vi "to8bits.vi"(2 "error in (no error)":errorcluster, 3 "Image":T1) -> (0 "error out":errorcluster, 1 "Image":T1)   [LabVIEW 2009]
uses:
  <vilib>/vision/Image Controls.llb/IMAQ Image.ctl
  <vilib>/vision/NI_Vision_Development_Module.lvlib
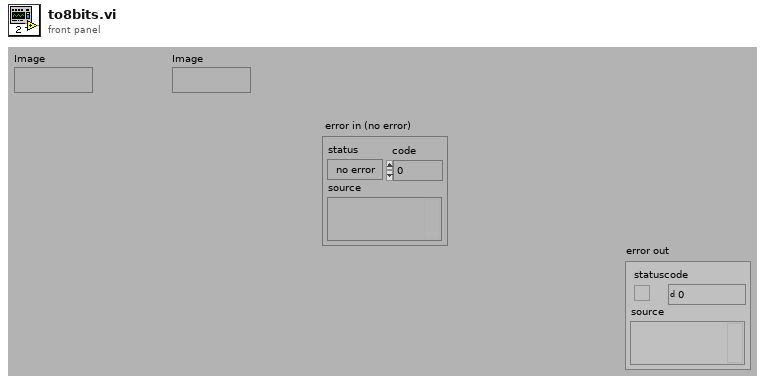
[diagram p1: front panel]
types:
  T1 = typedef "IMAQ Image.ctl" = refnum<image>
  T2 = cluster{"Mean Value":sgl, "Standard Variation":sgl, "Minimal Value":sgl, "Maximal Value":sgl, "Area (calibrated)":sgl, "Area (pixels)":i32, "%":sgl}
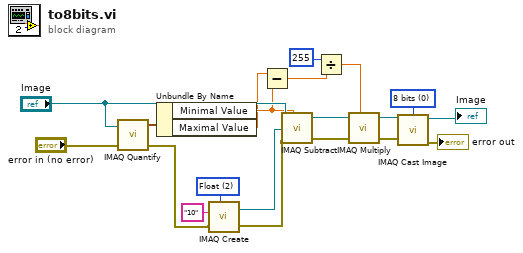
[diagram p0: block diagram]
diagram:
  w8 = u32 2 items=["8 bits", "16 bits", "Float", "Complex", "RGB", "HSL"] ("Image Type")
  w10 = u32 0 items=["8 bits", "16 bits", "Float", "Complex", "RGB", "HSL"] ("Image Type")
  n1 = call "IMAQ Quantify"("error in (no error)"="error in (no error)", "Image"="Image") -> ("error out"=w5:errorcluster, "Global Report"=w18:T2)  [unwired: 1 in, 1 out]
  n2 = Unbundle By Name(w18) -> ("Minimal Value"=w17:sgl, "Maximal Value"=w16:sgl)
  n3 = call "IMAQ Create"("Image Name"="10", "Image Type"=w8, "error in (no error)"=w5) -> ("New Image"=w7:T1, "error out"=w4:errorcluster)  [unwired: 2 in]
  n4 = Subtract(x=w16, y=w17) -> (x-y=w14:sgl)
  n5 = call "IMAQ Subtract"("Image Src A"="Image", "Constant"=w17, "Image Dst"=w7, "error in (no error)"=w4) -> ("Image Dst Out"=w13:T1, "error out"=w3:errorcluster)  [unwired: 3 in]
  n6 = Divide(x=u16 255, y=w14) -> (x/y=w12:sgl)
  n7 = call "IMAQ Multiply"("Image Src A"=w13, "Constant"=w12, "error in (no error)"=w3) -> ("Image Dst Out"=w11:T1, "error out"=w2:errorcluster)  [unwired: 4 in]
  n8 = call "IMAQ Cast Image"("Image Type"=w10, "error in (no error)"=w2, "Image Src"=w11) -> ("error out"=→"error out":errorcluster, "Image Dst Out"=→"Image":T1)  [unwired: 7 in]
